vi "KH7008 Set All Channels.vi"(8 "error in (no error)":errorcluster, 10 "Channel Params []":T1[](array[typedef]), 11 "VISA Refnum in":refnum<visa-resource-name>="COM1") -> (0 "error out":errorcluster, 2 "Ch Params [] out":T1[](array[typedef]), 3 "VISA Refnum out":refnum<visa-resource-name>)   [LabVIEW 2019, in "Inst.Krohn-Hite-7008.lvclass"]
uses:
  Inst.Krohn-Hite-7008.lvclass
  Typedefs/SetAll-Cluster.ctl
  Typedefs/Channel-Enum.ctl
  Typedefs/Gain-Enum.ctl
  Typedefs/Filter-Enum.ctl
  Typedefs/Shunt-Enum.ctl
  Typedefs/Coupling-Enum.ctl
  Typedefs/Input Configuration-Enum.ctl
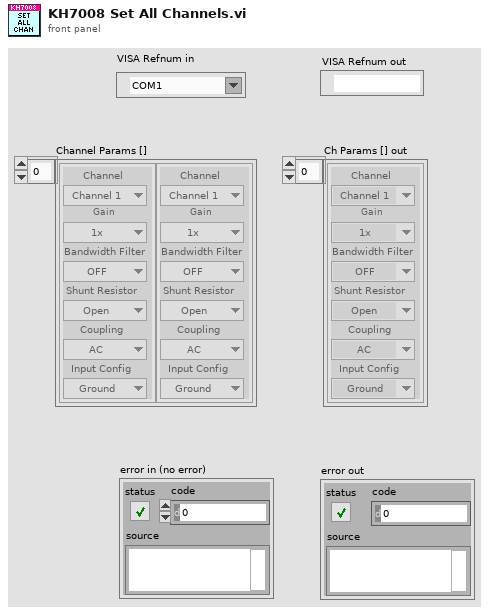
[diagram p1: front panel]
types:
  T1 = typedef "Inst.Krohn-Hite-7008.lvclass/SetAll-Cluster.ctl" = cluster{"Channel":T2, "Gain":T3, "Bandwidth Filter":T4, "Shunt Resistor":T5, "Coupling":T6, "Input Config":T7}
  T2 = typedef "Inst.Krohn-Hite-7008.lvclass/Channel-Enum.ctl" = enum16{"Channel 1", "Channel 2", "Channel 3", "Channel 4", "Channel 5", "Channel 6", "Channel 7", "Channel 8"}
  T3 = typedef "Inst.Krohn-Hite-7008.lvclass/Gain-Enum.ctl" = enum16{"1x", "10x", "100x", "1000x"}
  T4 = typedef "Inst.Krohn-Hite-7008.lvclass/Filter-Enum.ctl" = enum16{"OFF", "ON"}
  T5 = typedef "Inst.Krohn-Hite-7008.lvclass/Shunt-Enum.ctl" = enum16{"Open", "50 Ohms", "500 Ohms", "5k Ohms", "50k Ohms", "10M Ohm"}
  T6 = typedef "Inst.Krohn-Hite-7008.lvclass/Coupling-Enum.ctl" = enum16{"AC", "DC"}
  T7 = typedef "Inst.Krohn-Hite-7008.lvclass/Input Configuration-Enum.ctl" = enum16{"Ground", "SE+ (-gnd)", "SE- (+gnd)", "Differential"}
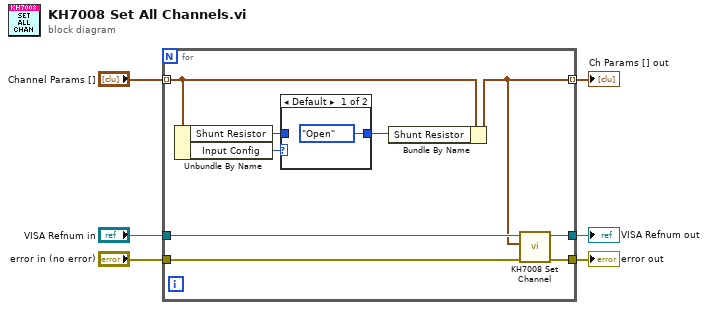
[diagram p0: block diagram]
diagram:
  n1 = for {
    tunnel: "Channel Params []" -> [w9] mode=indexing
    tunnel: [w7] -> w1 mode=indexing
    tunnel: "VISA Refnum in" -> [w14]
    tunnel: [w8] -> w2
    tunnel: "error in (no error)" -> [w11]
    tunnel: [w15] -> w4
    n2 = Unbundle By Name(w9) -> ("Shunt Resistor"=w13:T5, "Input Config"=w12:T7)
    n3 = case shown="Default" w12 {
      tunnel: [Shunt-Enum."Open" ("f") w17] -> w10
      tunnel: w13 -> [_ w17]
      frame Default {
      }
      frame "Differential" {
      }
    }
    n4 = Bundle By Name(cluster=w9, "Shunt Resistor"=w10) -> (w7:T1)
    n5 = call "KH7008 Set Channel.vi"("error in (no error)"=w11, "Channel Parameters"=w7, "VISA Refnum in"=w14) -> ("error out"=w15:errorcluster, "VISA Refnum out"=w8:refnum<visa-resource-name>)  [unwired: 7 in]
  }
  "error out" <- w4
  "VISA Refnum out" <- w2
  "Ch Params [] out" <- w1
